vi "set_up_KE6221.vi"(11 "VISA Refnum in":refnum<visa-resource-name>) -> (0 "error out":errorcluster, 3 "VISA Refnum out":refnum<visa-resource-name>, 5 "Check For SCPI Errors? (T)":bool)   [LabVIEW 2011]
uses:
  <instrlib>/Keithley 622x LV 2009/Utility/Typedefs/KE622x -- Instrument Type.ctl
  <instrlib>/Keithley 622x LV 2009/Typedefs/KE622x -- On Off Control.ctl
  <instrlib>/Keithley 622x LV 2009/Configure/Output/Typedefs/KE6221 -- Output Response.ctl
  <instrlib>/Keithley 622x LV 2009/Configure/Source/Typedefs/KE622x -- Current Range.ctl
  <instrlib>/Keithley 622x LV 2009/Configure/Source/Typedefs/KE622x -- Current Ranges.ctl
  <instrlib>/Keithley 622x LV 2009/Configure/Source/Typedefs/KE622x -- Voltage Limit.ctl
  <instrlib>/Keithley 622x LV 2009/Keithley 622x.lvlib
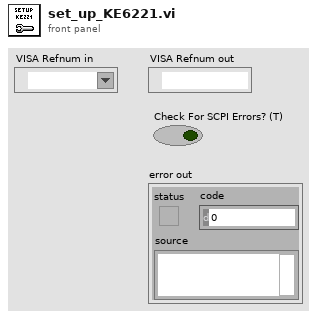
[diagram p1: front panel]
types:
  T1 = typedef "Keithley 622x.lvlib/KE622x -- On Off Control.ctl" = enum16{"Off", "On"}
  T2 = typedef "Keithley 622x.lvlib/KE622x -- Voltage Limit.ctl" = dbl
  T3 = typedef "Keithley 622x.lvlib/KE622x -- Current Range.ctl" = cluster{"Auto Range?":bool, "Man / Selected\nRange":T4}
  T4 = typedef "Keithley 622x.lvlib/KE622x -- Current Ranges.ctl" = enum16{"2nA", "20nA", "200nA", "2uA", "20uA", "200uA", "2mA", "20mA", "100mA"}
  T5 = typedef "Keithley 622x.lvlib/KE6221 -- Output Response.ctl" = enum16{"Fast", "Slow"}
  T6 = typedef "Keithley 622x.lvlib/KE622x -- Instrument Type.ctl" = enum16{"KE6220", "KE6221"}
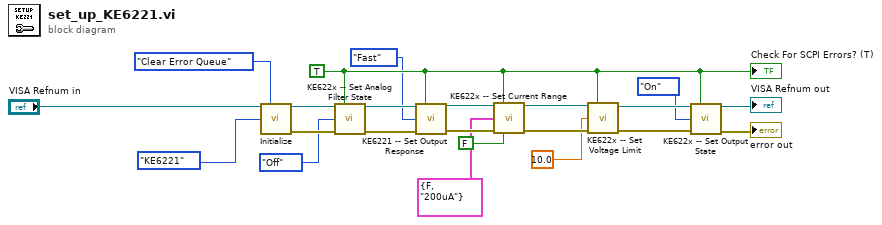
[diagram p0: block diagram]
diagram:
  w22 = TRUE ("Check For SCPI Errors? (T)")
  n1 = call <instrlib>:"Initialize.vi"("VISA resource name"="VISA Refnum in", "Error Queue Option"=enum16{"Clear Error Queue", "Error Query"}."Clear Error Queue", "Instrument Type"=KE622x_--_Instrument_Type."KE6221") -> ("VISA resource name out"=w4:refnum<visa-resource-name>, "error out"=w5:errorcluster)  [unwired: 11 in]
  n2 = call <instrlib>:"KE622x -- Set Analog Filter State.vi"("Resource In"=w4, "Check For SCPI Errors? (T)"=w22, "Analog Filter State"=KE622x_--_On_Off_Control."Off", "error in (no error)"=w5) -> ("Resource Out (dupl)"=w8:refnum<visa-resource-name>, "error out"=w9:errorcluster)  [unwired: 10 in]
  n3 = call <instrlib>:"KE6221 -- Set Output Response.vi"("Resource In"=w8, "Check For SCPI Errors? (T)"=w22, "KE6221 Output Response"=KE6221_--_Output_Response."Fast" ("Output Response"), "error in (no error)"=w9) -> ("Resource Out (dupl)"=w12:refnum<visa-resource-name>, "error out"=w13:errorcluster)  [unwired: 10 in]
  n4 = call <instrlib>:"KE622x -- Set Current Range.vi"("Resource In"=w12, "Check For SCPI Errors? (T)"=w22, "Current Range In"=T3 {"Auto Range?"=FALSE, "Man / Selected\nRange"=enum."200uA"}, "error in (no error)"=w13, "Read Back Set Values? (T)"=FALSE) -> ("Resource Out (dupl)"=w15:refnum<visa-resource-name>, "error out"=w16:errorcluster)  [unwired: 8 in, 1 out]
  n5 = call <instrlib>:"KE622x -- Set Voltage Limit.vi"("Resource In"=w15, "Check For SCPI Errors? (T)"=w22, "Voltage Limit (V)"=T2 10.0, "error in (no error)"=w16) -> ("Resource Out (dupl)"=w18:refnum<visa-resource-name>, "error out"=w19:errorcluster)  [unwired: 10 in]
  n6 = call <instrlib>:"KE622x -- Set Output State.vi"("Resource In"=w18, "Check For SCPI Errors? (T)"=w22, "Output State"=KE622x_--_On_Off_Control."On", "error in (no error)"=w19) -> ("Resource Out (dupl)"=→"VISA Refnum out":refnum<visa-resource-name>, "error out"=→"error out":errorcluster)  [unwired: 10 in]
  "Check For SCPI Errors? (T)" <- w22
